vi "shared-dependency-declareself&takeowner-test.vi"(8 "error in (no error)":errorcluster) -> (0 "error out":errorcluster)   [LabVIEW 2021]
uses:
  _test-support-SMOs/SMO.SelfTerminatingOverride/SMO.SelfTerminatingOverride.lvclass
  C:/Repositories/SMO/src/SMO/SMO.lvclass
  _test-support-SMOs/SMO.A/SMO.A.lvclass
  src/SMO/SMO.lvclass
  <vilib>/addons/_JKI Toolkits/Caraya/classes/Assert/Assert.lvclass
  <vilib>/addons/_JKI Toolkits/Caraya/classes/Test/Test.lvclass
  src/Registry/Registry-SMO.lvclass
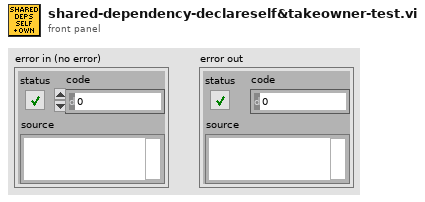
[diagram p1: front panel]
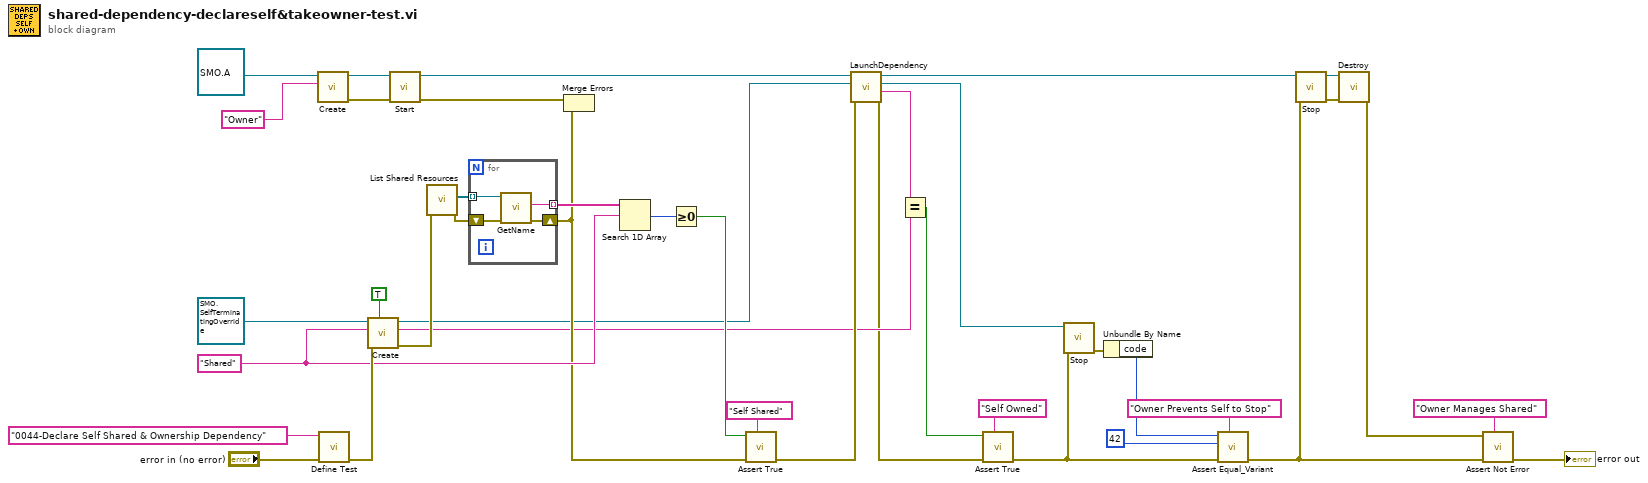
[diagram p0: block diagram]
diagram:
  w26 = "Shared" ("Subsystem Name (optional)")
  n1 = call "Create.vi"("Subsystem Name (optional)"="Owner", "SMO"=refnum<class "SMO.A.lvclass"> refnum ("SMO.A.lvclass")) -> ("error out"=w27:errorcluster, "SMO out"=w29:refnum<class "SMO.A.lvclass">)  [unwired: 7 in, 1 out]
  n2 = call <vilib>:"Define Test.vi"("error in (no error)"="error in (no error)", "Label (VI Title)"="0044-Declare Self Shared & Ownership Dependency") -> ("error out"=w36:errorcluster)  [unwired: 9 in]
  n3 = call "Create.vi"("Shared Resource (F)"=TRUE, "error in (no error)"=w36, "Subsystem Name (optional)"=w26, "SMO"=refnum<class "SMO.SelfTerminatingOverride.lvclass"> refnum ("SMO.SelfTerminatingOverride.lvclass")) -> ("error out"=w24:errorcluster, "SMO name"=w19:string, "SMO out"=w21:refnum<class "SMO.SelfTerminatingOverride.lvclass">)  [unwired: 5 in]
  n4 = call "Start.vi"("error in (no error)"=w27, "SMO"=w29) -> ("error out"=w23:errorcluster, "SMO out"=w25:refnum<class "SMO.A.lvclass">)  [unwired: 8 in]
  n5 = call "List Shared Resources.vi"("error in (no error)"=w24) -> ("error out"=w34:errorcluster, "Shared Resources"=w35:refnum<class "SMO.lvclass">[])  [unwired: 9 in]
  n6 = for {
    tunnel: w35 -> [w44] mode=indexing
    tunnel: [w43] -> w33 mode=indexing
    shift-right: [w41] -> w22
    shift-left: w34 -> [w42]
    n7 = call "GetName.vi"("error in (no error)"=w42, "SMO"=w44) -> ("error out"=w41:errorcluster, "Name"=w43:string)  [unwired: 6 in, 2 out]
  }
  n8 = Merge Errors(w23, w22) -> ()  [unwired: 1 out]
  n9 = Search 1D Array(1D array=w33, element=w26) -> (index of element=w32:i32)  [unwired: 1 in]
  n10 = Greater Or Equal To 0?(x=w32) -> (x >= 0?=w31:bool)
  n11 = call <vilib>:"Assert True.vi"("Label"="Self Shared" ("Filter (regex|name)"), "error in (no error)"=w22, "True?"=w31) -> ("error out"=w20:errorcluster)  [unwired: 8 in]
  n12 = call "LaunchDependency.vi"("error in (no error)"=w20, "Dependency Type"=w21, "SMO in"=w25) -> ("error out"=w15:errorcluster, "Unique Name"=w18:string, "Dependency Reference"=w8:refnum<class "SMO.SelfTerminatingOverride.lvclass">, "SMO out"=w14:refnum<class "SMO.A.lvclass">)  [unwired: 5 in]
  n13 = Equal?(x=w18, y=w19) -> (x = y?=w16:bool)
  n14 = call <vilib>:"Assert True.vi"("Label"="Self Owned" ("Filter (regex|name)"), "error in (no error)"=w15, "True?"=w16) -> ("error out"=w5:errorcluster)  [unwired: 8 in]
  n15 = call "Stop.vi"("error in (no error)"=w5, "SMO"=w8) -> ("error out"=w4:errorcluster)  [unwired: 8 in, 1 out]
  n16 = Unbundle By Name(w4) -> ("code"=w3:i32)
  n17 = call <vilib>:"Assert Equal_Variant.vi"("Label"="Owner Prevents Self to Stop" ("Filter (regex|name)"), "error in (no error)"=w5, "Y"=42 ("code"), "X"=w3) -> ("error out"=w6:errorcluster)  [unwired: 7 in]
  n18 = call "Stop.vi"("error in (no error)"=w6, "SMO"=w14) -> ("error out"=w12:errorcluster, "SMO out"=w13:refnum<class "SMO.A.lvclass">)  [unwired: 8 in]
  n19 = call "Destroy.vi"("error in (no error)"=w12, "SMO"=w13) -> ("error out"=w9:errorcluster)  [unwired: 9 in]
  n20 = call <vilib>:"Assert Not Error.vi"("Label"="Owner Manages Shared" ("Filter (regex|name)"), "error in (no error)"=w6, "Not Error?"=w9) -> ("error out"=→"error out":errorcluster)  [unwired: 8 in]
